vi "Move Channel Group.vi"(7 "Up (T) / Down (F)":bool, 8 "error in (no error)":errorcluster, 9 "ChanGroup":i32, 11 "TimingGrp in":refnum<class "TimingGrp.lvclass">) -> (0 "error out":errorcluster, 1 "ChanGroup Out":i32, 2 "Canceled?":bool, 3 "TimingGrp Out":refnum<class "TimingGrp.lvclass">)   [LabVIEW 2012, in "Configuration Grandmaster.lvlib" / "TimingGrp.lvclass"]
uses:
  TimingGrp.lvclass
  TimingGrp.lvclass/TimingGrp.ctl
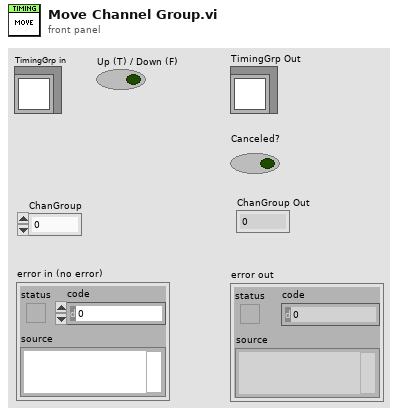
[diagram p1: front panel]
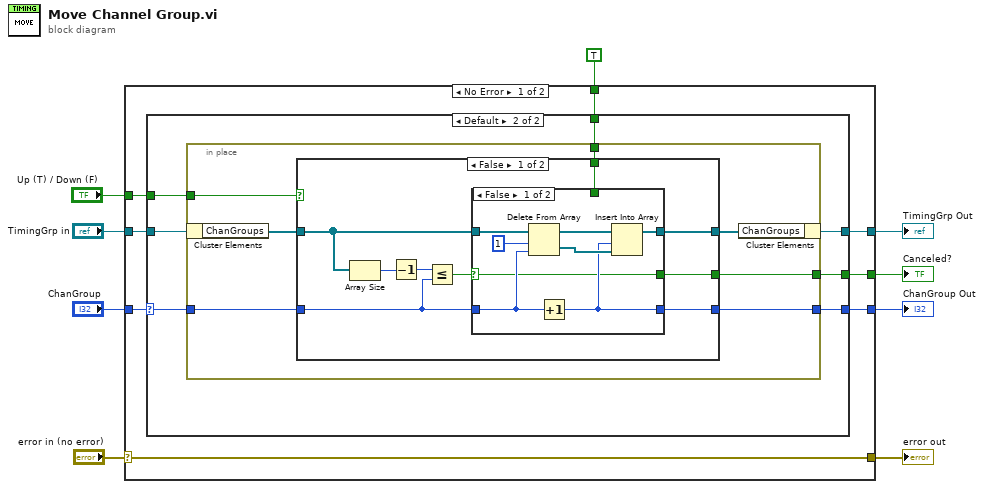
[diagram p0: block diagram]
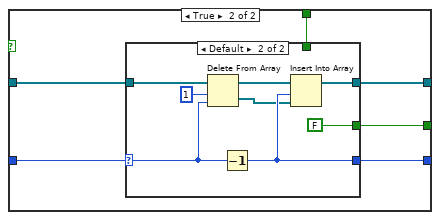
[diagram p4: hidden frame]
diagram:
  n1 = case shown="No Error" "error in (no error)" {
    selector: "error in (no error)" -> [w14 w74]
    tunnel: [w17 w75] -> w9
    tunnel: "ChanGroup" -> [w13 w75]
    tunnel: "TimingGrp in" -> [w16 w73]
    tunnel: [w15 w73] -> w6
    tunnel: [w14 w74] -> w4
    tunnel: [w12 w72] -> w3
    tunnel: TRUE -> [w11 w72]
    tunnel: "Up (T) / Down (F)" -> [w10 _]
    frame No Error {
      n2 = case shown="Default" w13 {
        selector: w13 -> [w19 w26]
        tunnel: [w19 w27] -> w17
        tunnel: w16 -> [w20 w25]
        tunnel: [w20 w24] -> w15
        tunnel: [w18 w22] -> w12
        tunnel: w11 -> [w18 w21]
        tunnel: w10 -> [_ w23]
        frame 0 {
        }
        frame Default {
          n3 = in-place {
            in-place-border: [w34] -> w27
            in-place-border: w26 -> [w33]
            in-place-border: w23 -> [w30]
            in-place-border: [w29] -> w22
            in-place-border: w21 -> [w28]
            n4 = in-place-cluster #1(w25) -> ("ChanGroups"=w32:refnum<class "ChanGrp.lvclass">[])
            n5 = case shown="False" w30 {
              tunnel: [w37 w60] -> w34
              tunnel: w33 -> [w38 w57]
              tunnel: w32 -> [w39 w59]
              tunnel: [w40 w58] -> w31
              tunnel: [w36 w56] -> w29
              tunnel: w28 -> [w35 w55]
              frame False {
                n6 = Array Size(array=w39) -> (size(s)=w42:i32)
                n7 = Decrement(x=w42) -> (x-1=w43:i32)
                n8 = Less Or Equal?(x=w43, y=w38) -> (x <= y?=w41:bool)
                n9 = case shown="False" w41 {
                  selector: w41 -> [w44 _]
                  tunnel: [w48 w53] -> w40
                  tunnel: [w47 w54] -> w37
                  tunnel: w39 -> [w46 w53]
                  tunnel: w38 -> [w45 w54]
                  tunnel: [w44 w52] -> w36
                  tunnel: w35 -> [_ w52]
                  frame False {
                    n10 = Delete From Array(array=w46, length=1, index=w45) -> (deleted portion=w50:refnum<class "ChanGrp.lvclass">[], array with subset deleted=w51:refnum<class "ChanGrp.lvclass">[])
                    n11 = Increment(x=w45) -> (x+1=w47:i32)
                    n12 = Insert Into Array(array=w51, index=w47, new element=w50) -> (w48:refnum<class "ChanGrp.lvclass">[])
                  }
                  frame True {
                  }
                }
              }
              frame True {
                n13 = case shown="Default" w57 {
                  selector: w57 -> [w62 w65]
                  tunnel: [w62 w71] -> w60
                  tunnel: w59 -> [w63 w67]
                  tunnel: [w63 w66] -> w58
                  tunnel: [w61 FALSE] -> w56
                  tunnel: w55 -> [w61 _]
                  frame 0 {
                  }
                  frame Default {
                    n14 = Delete From Array(array=w67, length=1, index=w65) -> (deleted portion=w69:refnum<class "ChanGrp.lvclass">[], array with subset deleted=w68:refnum<class "ChanGrp.lvclass">[])
                    n15 = Decrement(x=w65) -> (x-1=w71:i32)
                    n16 = Insert Into Array(array=w68, index=w71, new element=w69) -> (w66:refnum<class "ChanGrp.lvclass">[])
                  }
                }
              }
            }
            n17 = in-place-cluster #1("ChanGroups"=w31) -> (w24:refnum<class "TimingGrp.lvclass">)
          }
        }
      }
    }
    frame Error {
    }
  }
  "ChanGroup Out" <- w9
  "TimingGrp Out" <- w6
  "error out" <- w4
  "Canceled?" <- w3
